vi "LaunchProcess.vi"(8 "error in (no error)":errorcluster, 10 "ms timeout (1000)":i32=1000, 11 "obj":refnum<class "SimPump.lvclass">) -> (0 "error out":errorcluster, 3 "obj out":refnum<class "SimPump.lvclass">)   [LabVIEW 2019, in "SimPump.lvclass"]
doc: "Launches the active object process\n\nwww.sciware.com.au"
uses:
  SimPump.lvclass
  CmdQueueType.ctl
  MsgQueueType.ctl
  SimPump.lvclass/SimPump.ctl
panel:
  # "BSD License (http://www.opensource.org/licenses/bsd-license.php)"
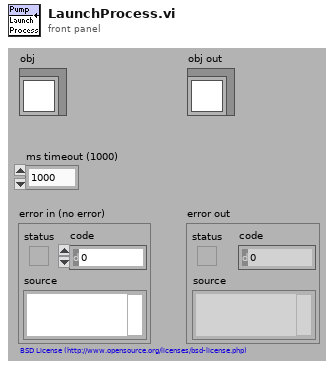
[diagram p1: front panel]
types:
  T1 = typedef "SimPump.lvclass/MsgQueueType.ctl" = string
  T2 = typedef "SimPump.lvclass/CmdQueueType.ctl" = string
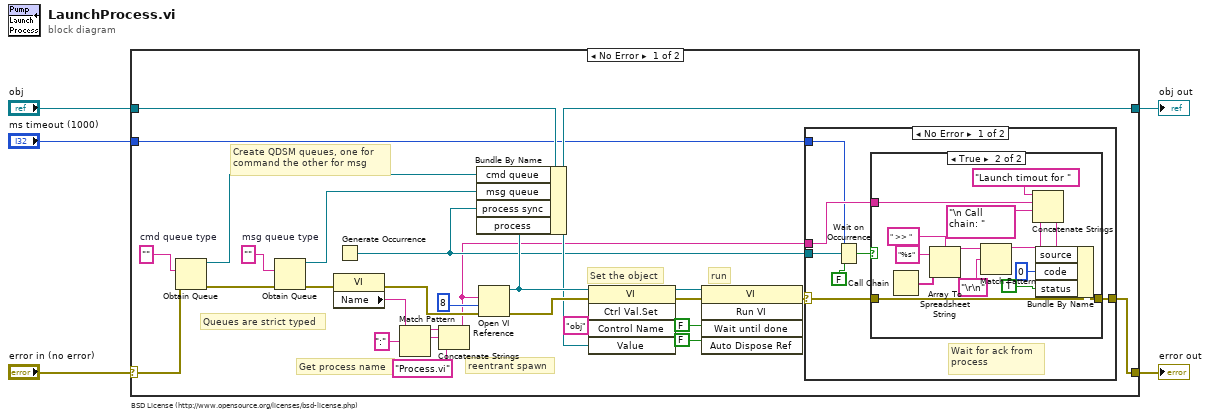
[diagram p0: block diagram]
diagram:
  # "BSD License (http://www.opensource.org/licenses/bsd-license.php)"
  n1 = case shown="No Error" "error in (no error)" {
    selector: "error in (no error)" -> [w33 w58]
    tunnel: [w10 w58] -> w4
    tunnel: [w13 w57] -> w2
    tunnel: "obj" -> [w27 w57]
    tunnel: "ms timeout (1000)" -> [w6 _]
    frame No Error {
      w30 = T1 ""  # msg queue type
      w32 = T2 ""  # cmd queue type
      # "run"
      # "Set the object"
      # "reentrant spawn"
      # "Get process name"
      # "Queues are strict typed"
      # "Create QDSM queues, one for\ncommand the other for msg"
      n2 = Obtain Queue(element data type=w32, error in (no error)=w33) -> (queue out=w29:refnum<queue>, error out=w31:errorcluster)  [unwired: 3 in, 1 out]
      n3 = Obtain Queue(element data type=w30, error in (no error)=w31) -> (queue out=w28:refnum<queue>, error out=w21:errorcluster)  [unwired: 3 in, 1 out]
      n4 = property class="VI"(error in=w21) -> (error out=w20:errorcluster, "Name"=w26:string)  [unwired: 1 in, 1 out]
      n5 = Generate Occurrence() -> (w11:refnum<k4>)
      n6 = Match Pattern(string=w26, regular expression=":") -> (before substring=w24:string, match substring=w23:string)  [unwired: 1 in, 2 out]
      n7 = Concatenate Strings(w24, w23, "Process.vi" ("string")) -> (w7:string)
      n8 = Open VI Reference(vi path=w7, options=8, error in (no error)=w20) -> (vi reference=w17:refnum<vi>, error out=w15:errorcluster)  [unwired: 3 in]
      n9 = Bundle By Name(cluster=w27, "cmd queue"=w29, "msg queue"=w28, "process sync"=w11, "process"=w17) -> (w13:refnum<class "SimPump.lvclass">)
      n10 = invoke class="VI" method="Ctrl Val.Set"(reference=w17, error in=w15, "Control Name"="obj", "Value"=w13) -> (reference out=w16:refnum<vi>, error out=w14:errorcluster)  [unwired: 1 in, 3 out]
      n11 = invoke class="VI" method="Run VI"(reference=w16, error in=w14, "Wait until done"=FALSE ("Wait Until Done"), "Auto Dispose Ref"=FALSE ("Auto Dispose Reference")) -> (error out=w8:errorcluster)  [unwired: 1 in, 4 out]
      n12 = case shown="No Error" w8 {
        selector: w8 -> [w36 w56]
        tunnel: w11 -> [w40 _]
        tunnel: [w39 w56] -> w10
        tunnel: w7 -> [w35 _]
        tunnel: w6 -> [w34 _]
        frame No Error {
          # "Wait for ack from\nprocess"
          n13 = Wait on Occurrence(1:FALSE ("ignore previous (T)"), 2:w40, 3:w34) -> (0:w37:bool)
          n14 = case shown="True" w37 {
            tunnel: w36 -> [w41 w44]
            tunnel: [w41 w43] -> w39
            tunnel: w35 -> [_ w42]
            frame False {
            }
            frame True {
              n15 = Call Chain() -> (call chain=w48:string[])
              n16 = Array To Spreadsheet String(delimiter (Tab)=" >> ", array=w48, 3:"%s" ("format string")) -> (spreadsheet string=w49:string)
              n17 = Match Pattern(string=w49, regular expression="\r\n") -> (before substring=w47:string)  [unwired: 4 out]
              n18 = Concatenate Strings("Launch timout for " ("source"), w42, "\n Call chain: " ("string"), w47) -> (w55:string)
              n19 = Bundle By Name(cluster=w44, "source"=w55, "code"=0, "status"=TRUE) -> (w43:errorcluster)
            }
          }
        }
        frame Error {
        }
      }
    }
    frame Error {
    }
  }
  "error out" <- w4
  "obj out" <- w2
